vi "sortItIntoArray.vi"(0 "element":u32, 1 "VoltArray":u32[](array[numeric]), 3 "actVoltIndex":i32, 4 "actScanIndex":i32, 5 "CounterArray":u32[][][](array[numeric]), 8 "actEventIndex":i32, 9 "nOfSteps":i32, 11 "TRSArrayIn":u32[][][](array[numeric])) -> (10 "actEventIndexOut":i32, 13 "TRSArrayOut":u32[][][](array[numeric]), 14 "VoltArrayOut":u32[](array[numeric]), 17 "actVoltIndexOut":i32, 18 "actScanIndexOut":i32, 19 "CounterArrayOut":u32[][][](array[numeric]))   [LabVIEW 2014]
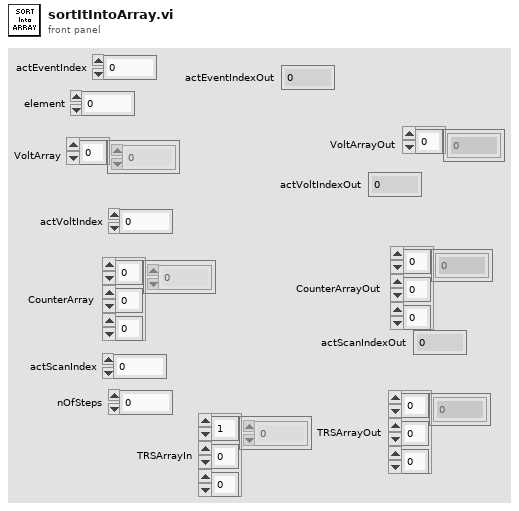
[diagram p1: front panel]
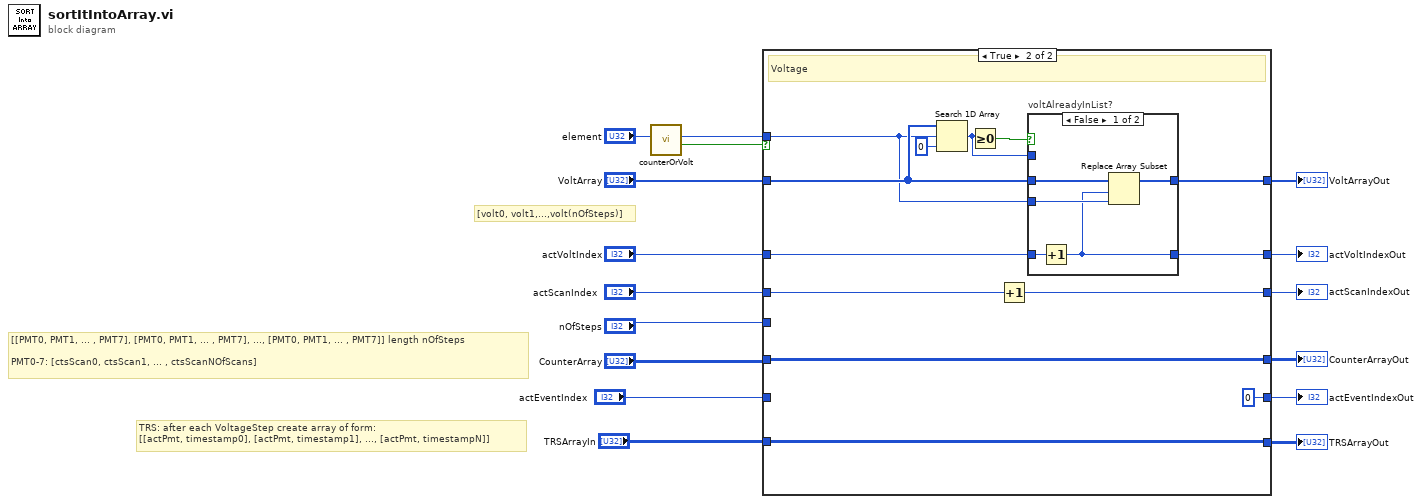
[diagram p0: block diagram]
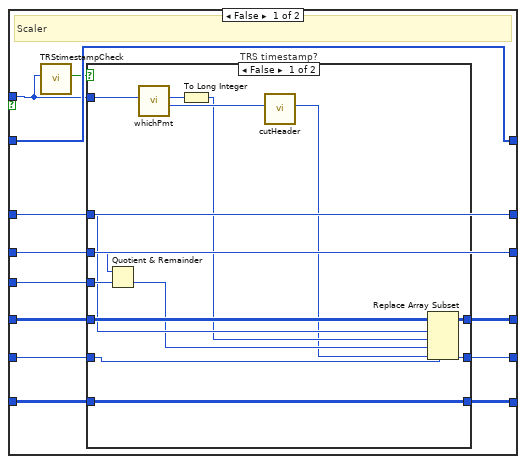
[diagram p2: hidden frame]
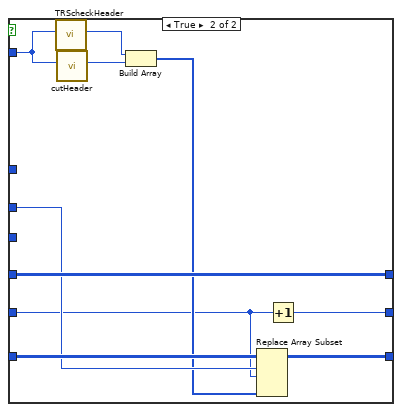
[diagram p3: hidden frame]
diagram:
  # "TRS: after each VoltageStep create array of form:\n[[actPmt, timestamp0], [actPmt, timestamp1], ..., [actPmt, timestampN]]"
  # "[[PMT0, PMT1, ... , PMT7], [PMT0, PMT1, ... , PMT7], ..., [PMT0, PMT1, ... , PMT7]] length nOfSteps\n\nPMT0-7: [ctsScan0, ctsScan1, ... , ctsScanNOfScans]"
  # "[volt0, volt1,...,volt(nOfSteps)]"
  n1 = call "counterOrVolt.vi"("element"="element") -> ("volt"=w5:bool, "elementOut"=w14:u32)  [unwired: 9 in]
  n2 = case shown="True" w5 {
    tunnel: "VoltArray" -> [w28 w62]
    tunnel: w14 -> [w22 w58]
    tunnel: "actVoltIndex" -> [w24 w59]
    tunnel: [w28 w61] -> w13
    tunnel: "CounterArray" -> [w27 w60]
    tunnel: [w26 w60] -> w11
    tunnel: [w24 w57] -> w10
    tunnel: "actScanIndex" -> [w23 w55]
    tunnel: "nOfSteps" -> [w25 _]
    tunnel: [w23 w54] -> w7
    tunnel: "TRSArrayIn" -> [w20 w53]
    tunnel: [w19 w53] -> w3
    tunnel: "actEventIndex" -> [w18 _]
    tunnel: [w17 0 ("actEventIndex")] -> w1
    frame False {
      # "Scaler"
      n3 = call "TRStimestampCheck.vi"("element"=w22) -> ("TRSTimestamp?"=w21:bool)  [unwired: 10 in]
      n4 = case "TRS timestamp?" shown="False" w21 {
        tunnel: w22 -> [w41 w50]
        tunnel: w27 -> [w39 w51]
        tunnel: [w38 w51] -> w26
        tunnel: w25 -> [w36 _]
        tunnel: w24 -> [w35 _]
        tunnel: w23 -> [w34 w47]
        tunnel: w20 -> [w30 w48]
        tunnel: [w30 w49] -> w19
        tunnel: w18 -> [w29 w43]
        tunnel: [w29 w42] -> w17
        frame False {
          n5 = Quotient & Remainder(x=w34, y=w36) -> (floor(x/y)=w32:i32)  [unwired: 1 out]
          n6 = call "whichPmt.vi"("element"=w41) -> ("elementOut"=w37:u32, "pmtNumber"=w40:u32)  [unwired: 9 in]
          n7 = To Long Integer(number=w40) -> (32bit integer=w33:i32)
          n8 = call "cutHeader.vi"("element"=w37) -> ("elementwithoutHeader"=w31:u32)  [unwired: 10 in]
          n9 = Replace Array Subset(array=w39, new element=w31, index (dim 0)=w35, index (dim 1)=w33, index (dim 2)=w32) -> (w38:u32[][][])
        }
        frame True {
          n10 = call "TRScheckHeader.vi"("element"=w50) -> ("actPmts"=w46:u32)  [unwired: 10 in]
          n11 = call "cutHeader.vi"("element"=w50) -> ("elementwithoutHeader"=w45:u32)  [unwired: 10 in]
          n12 = Build Array(w46, w45) -> (w44:u32[])
          n13 = Replace Array Subset(array=w48, new element=w44, index (dim 0)=w47, index (dim 1)=w43) -> (w49:u32[][][])  [unwired: 1 in]
          n14 = Increment(x=w43) -> (x+1=w42:i32)
        }
      }
    }
    frame True {
      # "Voltage"
      n15 = Search 1D Array(1D array=w62, element=w58, start index (0)=0) -> (index of element=w56:i32)
      n16 = Greater Or Equal To 0?(x=w56) -> (x >= 0?=w63:bool)
      n17 = Increment(x=w55) -> (x+1=w54:i32)
      n18 = case "voltAlreadyInList?" shown="False" w63 {
        tunnel: w62 -> [w69 w71]
        tunnel: [w68 w71] -> w61
        tunnel: w59 -> [w66 _]
        tunnel: w58 -> [w67 _]
        tunnel: [w65 w70] -> w57
        tunnel: w56 -> [_ w70]
        frame False {
          n19 = Increment(x=w66) -> (x+1=w65:i32)
          n20 = Replace Array Subset(array=w69, new element=w67, index=w65) -> (w68:u32[])
        }
        frame True {
        }
      }
    }
  }
  "VoltArrayOut" <- w13
  "CounterArrayOut" <- w11
  "actVoltIndexOut" <- w10
  "actScanIndexOut" <- w7
  "TRSArrayOut" <- w3
  "actEventIndexOut" <- w1
